vi "Analog Write Multiple.vi"(8 "error in (no error)":errorcluster, 10 "Analog Data":dbl[](array[numeric]), 11 "Analog Writer in":refnum<class "Analog Writer.lvclass">) -> (0 "error out":errorcluster, 3 "Analog Writer out":refnum<class "Analog Writer.lvclass">)   [LabVIEW 2024, in "DAQmx Actor.lvlib" / "Analog Writer.lvclass"]
uses:
  Analog Writer.lvclass
  <vilib>/DAQmx/write.llb/DAQmx Write (Analog 1D DBL NChan 1Samp).vi
  <vilib>/DAQmx/miscellaneous.llb/DAQmx Fill In Error Info.vi
  Analog Writer.lvclass/Analog Writer.ctl
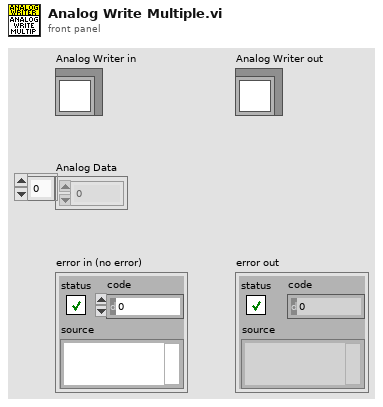
[diagram p1: front panel]
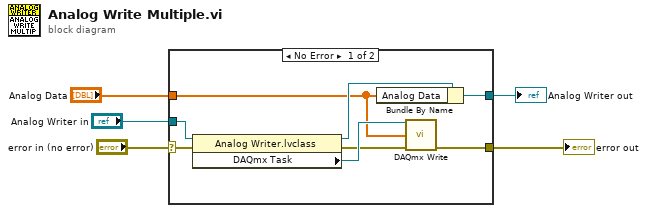
[diagram p0: block diagram]
diagram:
  n1 = case shown="No Error" "error in (no error)" {
    selector: "error in (no error)" -> [w9 w15]
    tunnel: [w10 w15] -> w4
    tunnel: [w6 w14] -> w2
    tunnel: "Analog Writer in" -> [w13 w14]
    tunnel: "Analog Data" -> [w7 _]
    frame No Error {
      n2 = property class="Analog Writer.lvclass"(reference=w13, error in=w9) -> (reference out=w8:refnum<class "Analog Writer.lvclass">, error out=w11:errorcluster, "DAQmx Task"=w12:refnum<k21>)
      n3 = Bundle By Name(cluster=w8, "Analog Data"=w7) -> (w6:refnum<class "Analog Writer.lvclass">)
      n4 = call-poly <vilib>:"DAQmx Write.vi"("task/channels in"=w12, "data"=w7, "error in"=w11) -> ("error out"=w10:errorcluster)  [unwired: 10 in, 2 out]
    }
    frame Error {
    }
  }
  "error out" <- w4
  "Analog Writer out" <- w2
